vi "Robot Global Data.vi"() -> ()   [LabVIEW 2020]
doc: "This global VI can contain as many global variables as you need. Place a control on the panel, give it a good name. To read or write to it from a VI, drag the icon to the diagram of that VI. You can also drag from the project. Click on the node to change which global you access. You shouldn't have multiple locations writing to a global or it will cause a race-condition."
uses:
  <vilib>/Rock Robotics/WPI/Camera/WPI_CameraImageSize.ctl
  <vilib>/Rock Robotics/WPI/DriverStation/WPI_DriverStationRobotMode2.ctl
panel:
  in  "Tab Control":T1(tab)
  in  "ALT":bool
  in  "JOY1 V P2":dbl
  in  "BTN RB":bool
  in  "BTN LB":bool
  in  "PAD":dbl
  in  "BTN X":bool
  in  "BTN Y":bool
  in  "BTN B":bool
  in  "BTN A":bool
  in  "JOY2 V":dbl
  in  "JOY2 H":dbl
  in  "GAT D":dbl
  in  "GAT E":dbl
  in  "JOY1 V":dbl
  in  "JOY1 H":dbl
  in  "ITK SUP MVT FC":bool
  in  "ITK MVT SUP ENC":dbl
  in  "ITK SUP CLT I":dbl
  in  "CHASSI MD ENC RST":bool
  in  "ACL YAW RST":bool
  in  "ITK INF MVT FC":bool
  in  "CHASSI MD ENC":dbl
  in  "ITK MVT INF ENC":dbl
  in  "ITK INF CLT I":dbl
  in  "ACL YAW":dbl
  in  "ACL ROLL":dbl
  in  "ACL PITCH":dbl
  in  "AUTO_CHARGE":bool
  in  "CORRIGE ITK SUP":bool
  in  "AUTO_CLT _INF":bool
  in  "AUTO_CLT_SUP":bool
  in  "AUTO_FREIO":bool
  in  "AUTO_MODE":bool
  in  "MVT INF AUTO":bool
  in  "ITK INF AUTO":bool
  in  "SERVO CTR":bool
  in  "CUBE DPT SUP":bool
  in  "CUBE ITK SUP":bool
  in  "CHASSI BREAK":bool
  in  "CUBE DPT INF":bool
  in  "CUBE ITK INF":bool
  in  "PIPELINE SLC":dbl
  in  "LIME ALINHAMENTO":bool
  out "LIME_AJUSTE_FINO":dbl
  out "LIME_AJUSTE_BRUTO":dbl
  out "LIME_LED":dbl
  out "LIME_TX":dbl
  in  "Robot Mode":T2
  in  "image size":T3=enum."320x240"
  in  "Enable Vision":bool
  # "0"
  # "0"
  # "1"
  # "1"
  # "1"
  # "-1"
  # "1"
  # "-1"
  # "-1"
  # "-1"
  # "1"
  # "1"
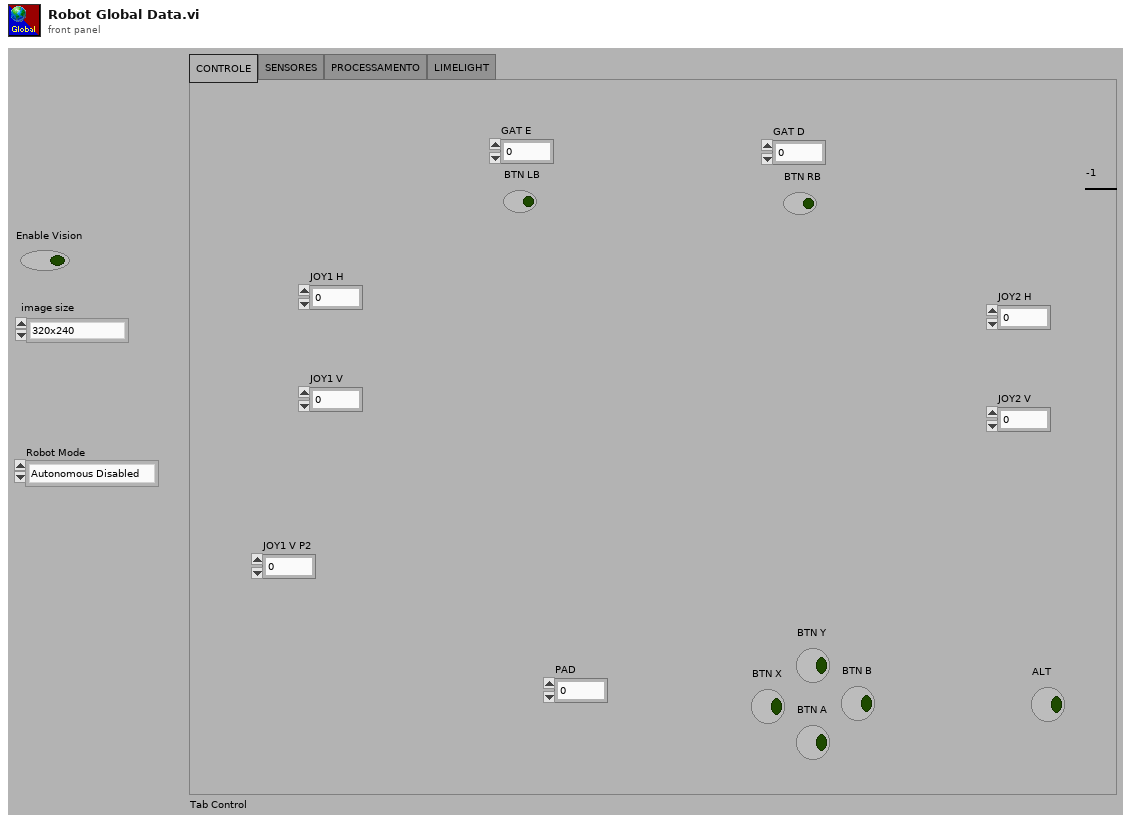
[diagram p1: front panel]
types:
  T1 = enum32{"CONTROLE", "SENSORES", "PROCESSAMENTO", "LIMELIGHT"}
  T2 = typedef "WPI_DriverStationRobotMode2.ctl" = enum16{"Autonomous Disabled", "Autonomous Enabled", "Teleop Disabled", "Teleop Enabled", "Disconnected", "Finish", "Test Disabled", "Test Enabled", "Emergency Stopped"}
  T3 = typedef "WPI_CameraImageSize.ctl" = enum16{"640x480", "320x240", "160x120", "Custom"}
diagram:
